vi "UDP_Send.vi"() -> ()   [LabVIEW 2017]
panel:
  out "connection ID out":refnum<k16>
  in  "connection ID":refnum<k16>
  out "字符串":string
  out "error out":errorcluster={"status"=TRUE, "code"=56, "source"="UDP Read in UDP.vi->flash.vi"}
  in  "error in (no error)":errorcluster
  out "Out":u8 format="%.0x"
  in  "In":u8=255 format="%.0x"
  in  "Read (TRUE)":bool
  in  "Address":u32=64 format="%.0x"
  in  "IP address":string="192.168.10.20"
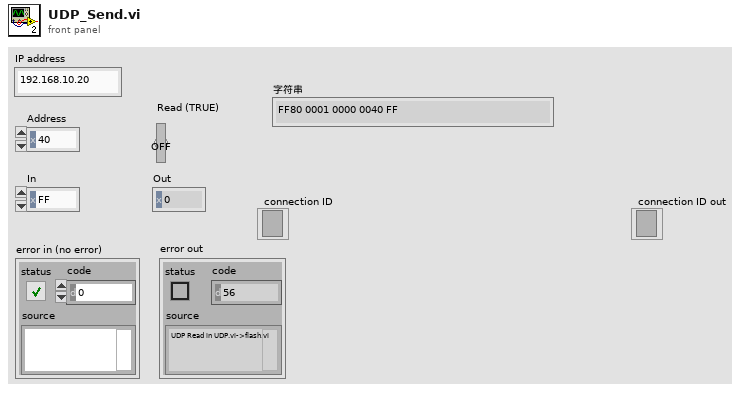
[diagram p1: front panel]
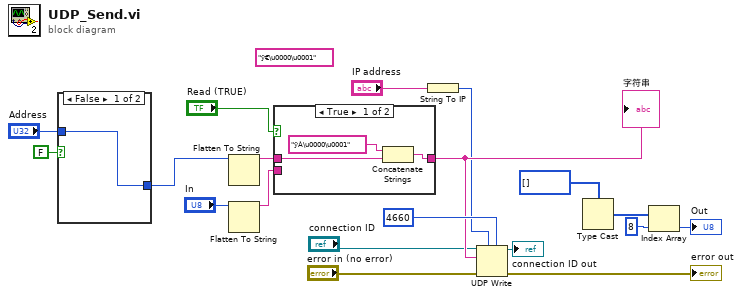
[diagram p0: block diagram]
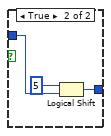
[diagram p2: hidden frame]
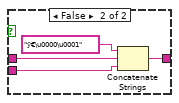
[diagram p3: hidden frame]
diagram:
  (unwired) "ÿ€\u0000\u0001" ("initial string")
  n1 = case shown="False" FALSE {
    tunnel: [w20 w22] -> w7
    tunnel: "Address" -> [w20 w21]
    frame False {
    }
    frame True {
      n2 = Logical Shift(y=i16 5, x=w21) -> (x << y=w22:u32)
    }
  }
  n3 = Flatten To String(anything=w7) -> (data string=w16:string)  [unwired: 3 in, 2 out]
  n4 = Flatten To String(anything="In") -> (data string=w14:string)  [unwired: 3 in, 2 out]
  n5 = case shown="True" "Read (TRUE)" {
    tunnel: [w25 w29] -> w17
    tunnel: w16 -> [w24 w28]
    tunnel: w14 -> [_ w27]
    frame True {
      n6 = Concatenate Strings("ÿÀ\u0000\u0001" ("initial string"), w24) -> (w25:string)
    }
    frame False {
      n7 = Concatenate Strings("ÿ€\u0000\u0001" ("initial string"), w28, w27) -> (w29:string)
    }
  }
  "字符串" <- w17
  n8 = String To IP(1:"IP address") -> (0:w8:u32)
  n9 = UDP Write(address=w8, port or service name=u16 4660 ("UDP port"), connection ID="connection ID", data in=w17, 8:"error in (no error)") -> (error out=→"error out":errorcluster, 3:→"connection ID out":refnum<k16>)  [unwired: 1 in]
  n10 = Type Cast(type=u8[] []) -> (*(type *) &x=w11:u8[])  [unwired: 1 in]
  n11 = Index Array(array=w11, index=8) -> (element=→"Out":u8)
